vi "SerialGlobal.vi"() -> ()   [LabVIEW 2018]
panel:
  in  "Key":string
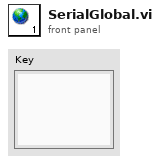
[diagram p1: front panel]
diagram:
